vi "FVIR_LDO_Ultramat_23.vi"(8 "error in":errorcluster, 10 "VISA resource name":refnum<visa-resource-name>="OXYMAT", 11 "Message Queues":T1) -> (0 "error out":errorcluster)   [LabVIEW 2020]
uses:
  Message Queue/All Message Queues.ctl
  Message Queue/Message Cluster.ctl
  Message Queue/Enqueue Message (Single).vi
  Message Queue/Message Queue.lvlib
panel:
  out "Loop Count":i32
  out "Gas Type":string
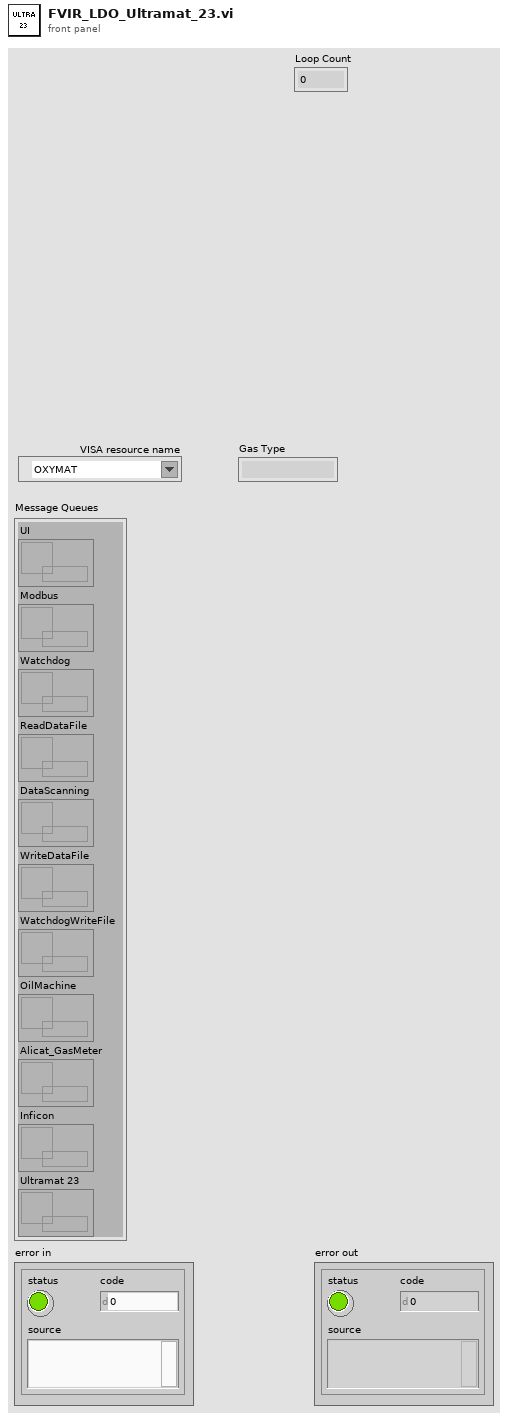
[diagram p1: front panel]
types:
  T1 = typedef "Message Queue.lvlib/All Message Queues.ctl" = cluster{"UI":refnum<queue>, "Modbus":refnum<queue>, "Watchdog":refnum<queue>, "ReadDataFile":refnum<queue>, "DataScanning":refnum<queue>, "WriteDataFile":refnum<queue>, "WatchdogWriteFile":refnum<queue>, "OilMachine":refnum<queue>, "Alicat_GasMeter":refnum<queue>, "Inficon":refnum<queue>, "Ultramat 23":refnum<queue>}
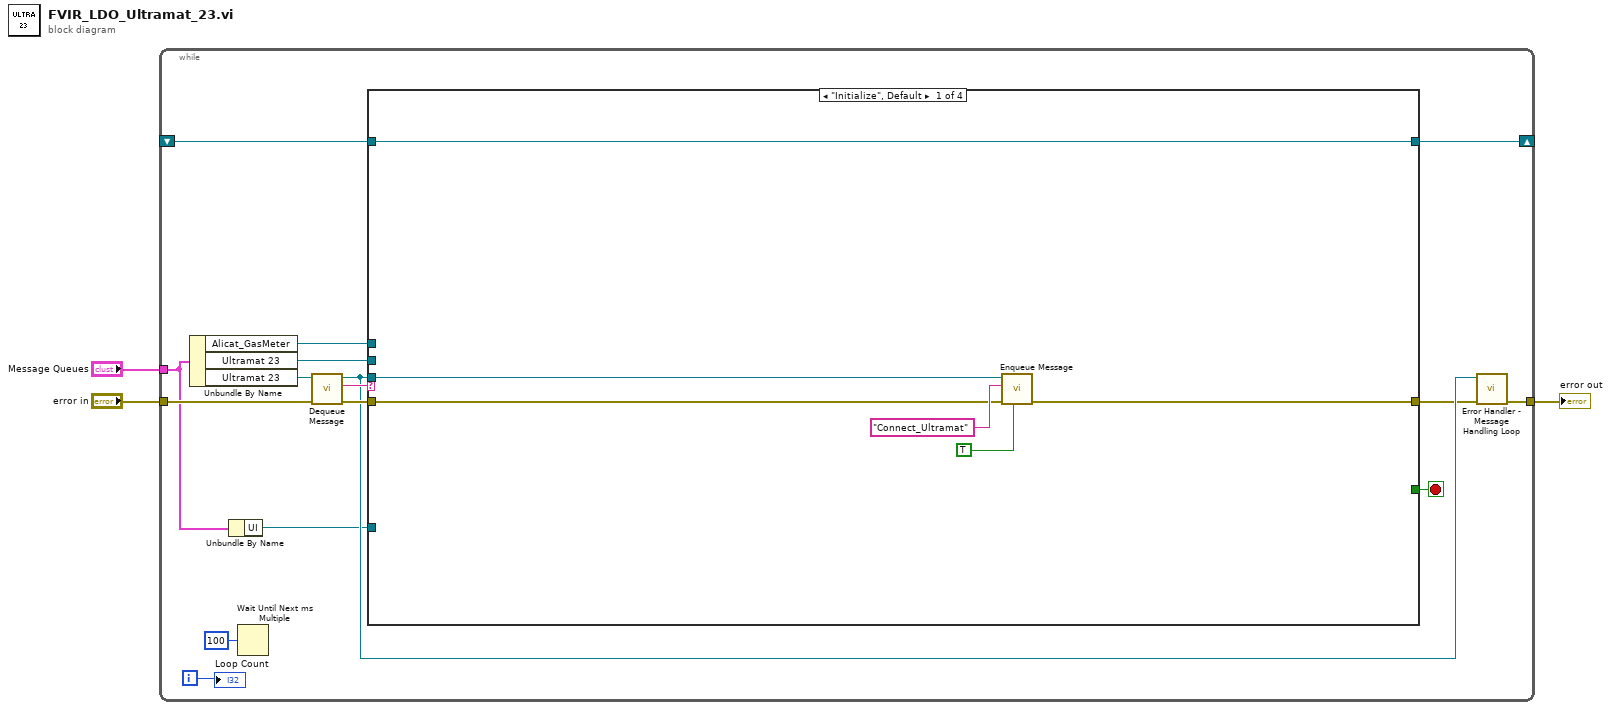
[diagram p0: block diagram]
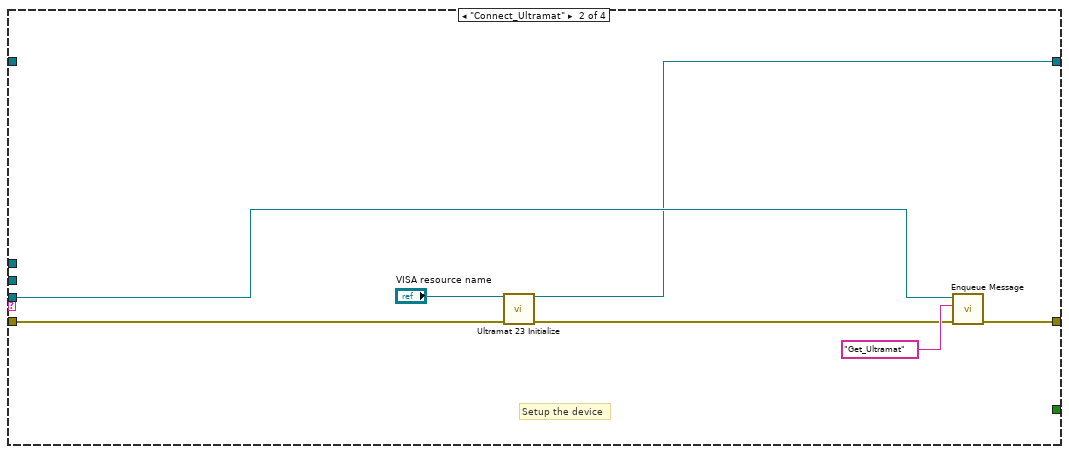
[diagram p2: hidden frame]
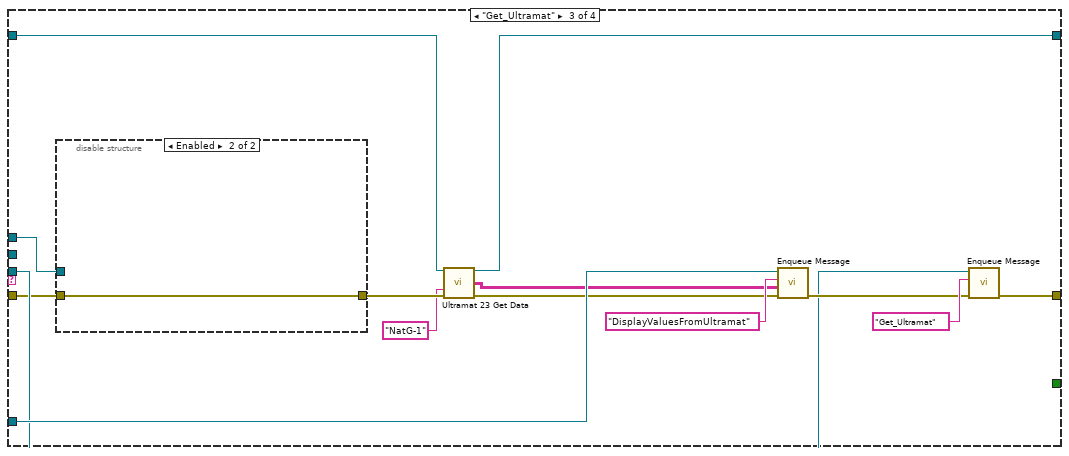
[diagram p3: hidden frame]
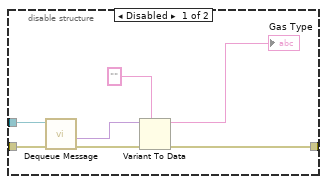
[diagram p4: hidden frame]
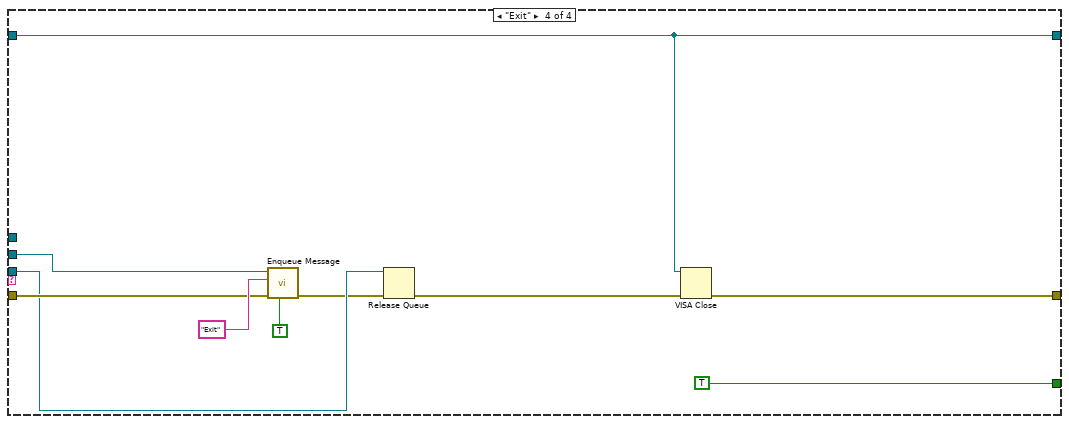
[diagram p5: hidden frame]
diagram:
  n1 = while {
    tunnel: "Message Queues" -> [w9]
    tunnel: "error in" -> [w18]
    tunnel: [w12] -> w1
    shift-right: [w7] -> _
    shift-left: _ -> [w6]
    i -> [w4]
    stop <- w15 stop-if-true
    n2 = Unbundle By Name(w9) -> ("Alicat_GasMeter"=w5:refnum<queue>, "Ultramat 23"=w14:refnum<queue>, "Ultramat 23"=w19:refnum<queue>)
    n3 = Unbundle By Name(w9) -> ("UI"=w8:refnum<queue>)
    n4 = Wait Until Next ms Multiple(millisecond multiple=u32 100) -> ()  [unwired: 1 out]
    n5 = call "Dequeue Message.vi"("error in (no error)"=w18, "Message Queue"=w19) -> ("error out"=w16:errorcluster, "Message"=w17:string, "dup Message Queue"=w13:refnum<queue>)  [unwired: 6 in, 1 out]
    n6 = case shown="\"Initialize\", Default" w17 {
      tunnel: w16 -> [w24 w29 w36 w60]
      tunnel: [w23 w31 w42 w56] -> w11
      tunnel: [_ _ _ TRUE] -> w15
      tunnel: w14 -> [_ _ _ w61]
      tunnel: w13 -> [w22 w30 w41 w59]
      tunnel: w8 -> [_ _ w45 _]
      tunnel: [w21 w26 w38 w55] -> w7
      tunnel: w6 -> [w21 _ w39 w55]
      tunnel: w5 -> [_ _ w35 _]
      frame "Initialize", Default {
        n7 = call-poly "Enqueue Message.vi"("Priority Message? (F)"=TRUE, "error in (no error)"=w24, "Message"="Connect_Ultramat", "Message Queue"=w22) -> ("error out"=w23:errorcluster)  [unwired: 6 in, 1 out]
      }
      frame "Connect_Ultramat" {
        # "Setup the device"
        n8 = call "Ultramat 23 Initialize.vi"("VISA resource name"="VISA resource name", "error in (no error)"=w29) -> ("VISA Session Out"=w26:refnum<visa-resource-name>, "error out"=w28:errorcluster)  [unwired: 8 in, 4 out]
        n9 = call-poly "Enqueue Message.vi"("error in (no error)"=w28, "Message"="Get_Ultramat", "Message Queue"=w30) -> ("error out"=w31:errorcluster)  [unwired: 7 in, 1 out]
      }
      frame "Get_Ultramat" {
        n10 = disable-structure shown="Enabled" {
          disable-tunnel: w36 -> [w53 w54]
          disable-tunnel: w35 -> [w52 _]
          disable-tunnel: [w48 w54] -> w34
          frame Disabled {
            n11 = call "Dequeue Message.vi"("error in (no error)"=w53, "Message Queue"=w52) -> ("error out"=w51:errorcluster, "Message Data"=w49:variant)  [unwired: 6 in, 2 out]
            n12 = Variant To Data(error in=w51, type="", Variant=w49) -> (data=→"Gas Type":string, error out=w48:errorcluster)
          }
          frame Enabled {
          }
        }
        n13 = call "Ultramat 23 Get Data.vi"("VISA resource name"=w39, "Gas selected"="NatG-1", "error in (no error)"=w34) -> ("VISA Session Out"=w38:refnum<visa-resource-name>, "Data Array"=w37:string[][], "error out"=w40:errorcluster)  [unwired: 8 in, 2 out]
        n14 = call-poly "Enqueue Message.vi"("error in (no error)"=w40, "Message Data"=w37, "Message"="DisplayValuesFromUltramat", "Message Queue"=w45) -> ("error out"=w43:errorcluster)  [unwired: 6 in, 1 out]
        n15 = call-poly "Enqueue Message.vi"("error in (no error)"=w43, "Message"="Get_Ultramat", "Message Queue"=w41) -> ("error out"=w42:errorcluster)  [unwired: 7 in, 1 out]
      }
      frame "Exit" {
        n16 = call-poly "Enqueue Message.vi"("Priority Message? (F)"=TRUE, "error in (no error)"=w60, "Message"="Exit", "Message Queue"=w61) -> ("error out"=w58:errorcluster)  [unwired: 6 in, 1 out]
        n17 = Release Queue(queue=w59, error in (no error)=w58) -> (error out=w57:errorcluster)  [unwired: 1 in, 2 out]
        n18 = VISA Close(VISA resource name=w55, error in (no error)=w57) -> (error out=w56:errorcluster)
      }
    }
    n19 = call "Error Handler - Message Handling Loop.vi"("error in (no error)"=w11, "Message Queue"=w13) -> ("dup error in"=w12:errorcluster)  [unwired: 8 in, 1 out]
    "Loop Count" <- w4
  }
  "error out" <- w1
